vi "Fetch Multi Eval Meas List Segment IEM Margin Results.vi"(6 "Segment (1)":T3=1, 8 "error in (no error)":errorcluster, 9 "Result Type (Current)":i32(ring) items=["Current", "Average", "Extreme", "Standard Deviation"], 10 "Instance (1)":T4=1, 11 "VISA resource name":refnum<visa-resource-name>) -> (0 "error out":errorcluster, 1 "Margin Results":T1 {"Carrier Leakage" format="%^.3e"; "IQ Image" format="%^.3e"; "Margin" format="%^.3e"}, 2 "Reliability":T2, 3 "VISA resource name out":refnum<visa-resource-name>, 4 "Expired Statistics":i32, 5 "Out Of Tolerance":i32)   [LabVIEW 2020, in "Rohde&Schwarz CMWXP NR FR1 Measurement.lvlib"]
doc: "Return the inband emission limit line margin results for segment <no> in list mode. The current margins indicate the minimum (vertical) distance between the limit line and the current trace. A negative result indicates that the limit is exceeded. The average, extreme and standard deviation values are calculated from the current margins.\n\nAttributes:\nRSCMWXPNRFR1M_ATTR_FETCH_MULTI_EVAL_MEAS_LIST_SEGMENT_IEM_MARGIN_CURRENT_RESULTS\nRSCMWXPNRFR1M_ATTR_FETCH_MULTI_EVAL_MEAS_LIST_SEGMENT_IEM_MARGIN_AVERAGE_RESULTS\nRSCMWXPNRFR1M_ATTR_FETCH_MULTI_EVAL_MEAS_LIST_SEGMENT_IEM_MARGIN_EXTREME_RESULTS\nRSCMWXPNRFR1M_ATTR_FETCH_MULTI_EVAL_MEAS_LIST_SEGMENT_IEM_MARGIN_STANDARD_DEVIATION_RESULTS\n\nRemote-control commands:\nFETCh:NRSub:MEAS<i>:MEValuation:LIST:SEGMent<no>:IEMission:MARGin:CURRent?\nFETCh:NRSub:MEAS<i>:MEValuation:LIST:SEGMent<no>:IEMission:MARGin:AVERage?\nFETCh:NRSub:MEAS<i>:MEValuation:LIST:SEGMent<no>:IEMission:MARGin:EXTReme?\nFETCh:NRSub:MEAS<i>:MEValuation:LIST:SEGMent<no>:IEMission:MARGin:SDEViation?"
uses:
  <instrlib>/Rohde&Schwarz CMWXP NR FR1 Measurement/Rohde&Schwarz CMWXP NR FR1 Measurement.lvlib
  <instrlib>/Rohde&Schwarz CMWXP NR FR1 Measurement/Private/_Instance.ctl
  <instrlib>/Rohde&Schwarz CMWXP NR FR1 Measurement/Private/_Segment.ctl
  <instrlib>/Rohde&Schwarz CMWXP NR FR1 Measurement/Private/_SegReliability.ctl
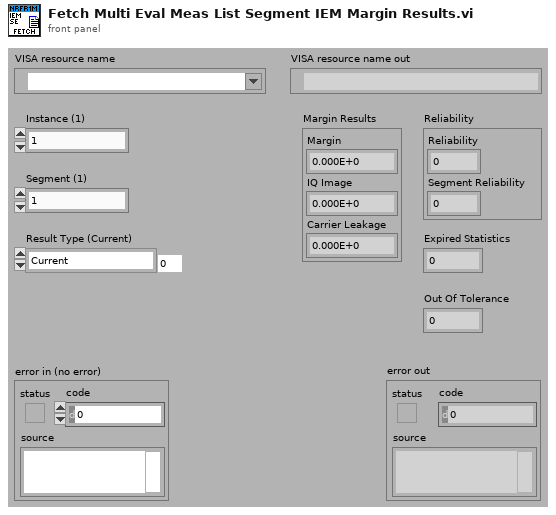
[diagram p1: front panel]
types:
  T1 = cluster{"Margin":dbl, "IQ Image":dbl, "Carrier Leakage":dbl}
  T2 = typedef "Rohde&Schwarz CMWXP NR FR1 Measurement.lvlib/_SegReliability.ctl" = cluster{"Reliability":i32, "Segment Reliability":i32}
  T3 = typedef "Rohde&Schwarz CMWXP NR FR1 Measurement.lvlib/_Segment.ctl" = i32
  T4 = typedef "Rohde&Schwarz CMWXP NR FR1 Measurement.lvlib/_Instance.ctl" = i32
  T5 = cluster{"Results[0]":dbl, "Results[1]":dbl, "Results[2]":dbl}
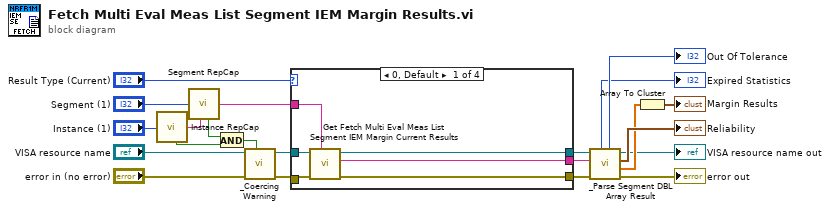
[diagram p0: block diagram]
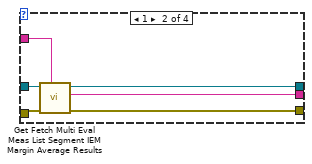
[diagram p2: hidden frame]
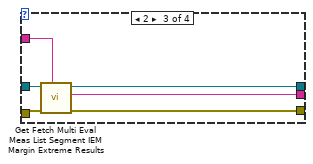
[diagram p3: hidden frame]
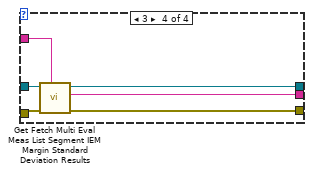
[diagram p4: hidden frame]
diagram:
  n1 = call <instrlib>:"Instance RepCap.vi"("Instance In"="Instance (1)") -> ("In Range?"=w19:bool, "RepCap Identifier Out"=w18:string)  [unwired: 1 in]
  n2 = call <instrlib>:"Segment RepCap.vi"("Segment In"="Segment (1)", "RepCap String In (\"\")"=w18) -> ("In Range?"=w17:bool, "RepCap Identifier Out"=w14:string)
  n3 = And(x=w17, y=w19) -> (x .and. y?=w16:bool)
  n4 = call <instrlib>:"_Coercing Warning.vi"("In Range?"=w16, "error in (no error)"="error in (no error)", "VISA resource name"="VISA resource name") -> ("error out"=w12:errorcluster, "VISA resource name out"=w13:refnum<visa-resource-name>)  [unwired: 7 in]
  n5 = case shown="0, Default" "Result Type (Current)" {
    tunnel: w14 -> [w28 w34 w40 w46]
    tunnel: w13 -> [w27 w33 w39 w45]
    tunnel: w12 -> [w26 w32 w38 w44]
    tunnel: [w25 w31 w37 w43] -> w8
    tunnel: [w24 w30 w36 w42] -> w9
    tunnel: [w23 w29 w35 w41] -> w10
    frame 0, Default {
      n6 = call "Get Fetch Multi Eval Meas List Segment IEM Margin Current Results"("Repeated Capabilities"=w28, "error in (no error)"=w26, "instrument handle"=w27) -> ("error out"=w23:errorcluster, "Fetch Multi Eval Meas List Segment IEM Margin Current Results"=w24:string, "instrument handle out"=w25:refnum<visa-resource-name>)  [unwired: 6 in]
    }
    frame 1 {
      n7 = call "Get Fetch Multi Eval Meas List Segment IEM Margin Average Results"("Repeated Capabilities"=w34, "error in (no error)"=w32, "instrument handle"=w33) -> ("error out"=w29:errorcluster, "Fetch Multi Eval Meas List Segment IEM Margin Average Results"=w30:string, "instrument handle out"=w31:refnum<visa-resource-name>)  [unwired: 6 in]
    }
    frame 2 {
      n8 = call "Get Fetch Multi Eval Meas List Segment IEM Margin Extreme Results"("Repeated Capabilities"=w40, "error in (no error)"=w38, "instrument handle"=w39) -> ("error out"=w35:errorcluster, "Fetch Multi Eval Meas List Segment IEM Margin Extreme Results"=w36:string, "instrument handle out"=w37:refnum<visa-resource-name>)  [unwired: 6 in]
    }
    frame 3 {
      n9 = call "Get Fetch Multi Eval Meas List Segment IEM Margin Standard Deviation Results"("Repeated Capabilities"=w46, "error in (no error)"=w44, "instrument handle"=w45) -> ("error out"=w41:errorcluster, "Fetch Multi Eval Meas List Segment IEM Margin Standard Deviation Results"=w42:string, "instrument handle out"=w43:refnum<visa-resource-name>)  [unwired: 6 in]
    }
  }
  n10 = call <instrlib>:"_Parse Segment DBL Array Result.vi"("error in (no error)"=w10, "Input String"=w9, "VISA resource name"=w8) -> ("error out"=→"error out":errorcluster, "Results"=w5:dbl[], "Reliability Results"=→"Reliability":T2, "VISA resource name out"=→"VISA resource name out":refnum<visa-resource-name>, "Out Of Tolerance"=→"Out Of Tolerance":i32, "Statistic Expired"=→"Expired Statistics":i32)  [unwired: 3 in]
  n11 = Array To Cluster(array=w5) -> (cluster=→"Margin Results":T5)
